vi "Alarm.FindEdittable.vi"(10 "String":string) -> (3 "Edit?":bool)   [LabVIEW 2015, in "Single Station Execution.lvlib"]
uses:
  Single Station Execution.lvlib
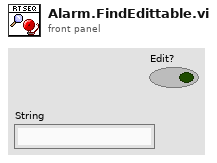
[diagram p1: front panel]
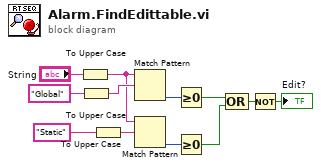
[diagram p0: block diagram]
diagram:
  n1 = To Upper Case(1:"String") -> (0:w2:string)
  n2 = To Upper Case(1:"Global" ("string")) -> (0:w6:string)
  n3 = To Upper Case(1:"Static" ("string")) -> (0:w9:string)
  n4 = Match Pattern(string=w2, regular expression=w6) -> (offset past match=w4:i32)  [unwired: 1 in, 3 out]
  n5 = Match Pattern(string=w2, regular expression=w9) -> (offset past match=w10:i32)  [unwired: 1 in, 3 out]
  n6 = Greater Or Equal To 0?(x=w4) -> (x >= 0?=w3:bool)
  n7 = Greater Or Equal To 0?(x=w10) -> (x >= 0?=w11:bool)
  n8 = Compound Arithmetic op=OR(w3, w11) -> (w12:bool)
  n9 = Not(x=w12) -> (.not. x?=→"Edit?":bool)
